vi "initialize Session Data.vi"(0 "Session in":refnum<class "SLSC Session.lvclass">, 11 "error in":errorcluster) -> (4 "Session out":refnum<class "SLSC Session.lvclass">, 15 "error out":errorcluster)   [LabVIEW 2015, in "SLSC Switch.lvlib" / "SLSC Session.lvclass"]
uses:
  SLSC Session.lvclass
  SLSC Session.lvclass/SLSC Session.ctl
  <vilib>/SLSC/Initialize Session without Resources.vi
  <userlib>/_Session Fwk/Session - Root.lvclass
  <vilib>/SLSC/SLSC.lvlib
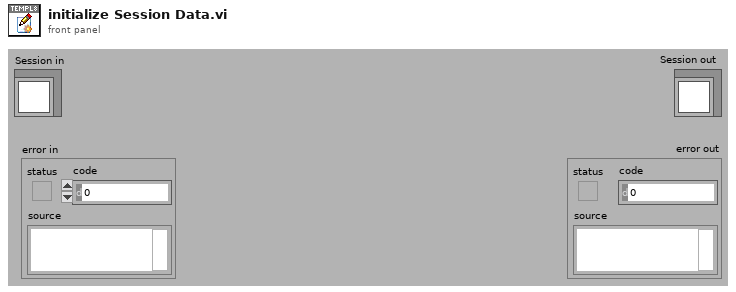
[diagram p1: front panel]
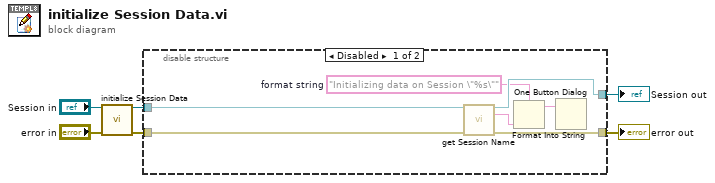
[diagram p0: block diagram]
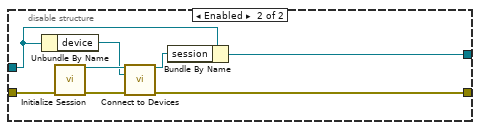
[diagram p2: hidden frame]
diagram:
  n1 = call-parent "initialize Session Data.vi"("OBJ - Session in"="Session in", "error in"="error in") -> ("OBJ - Session out"=w3:refnum<class "SLSC Session.lvclass">, "error out"=w1:errorcluster)  [unwired: 12 in]
  n2 = disable-structure shown="Disabled" {
    disable-tunnel: w3 -> [w13 w21]
    disable-tunnel: [w12 w20] -> w5
    disable-tunnel: w1 -> [w8 w15]
    disable-tunnel: [w7 w14] -> w6
    frame Disabled {
      w10 = "Initializing data on Session \"%s\""  # format string
      n3 = call <userlib>:"get Session Name.vi"("OBJ - Session in"=w13, "error in (no error)"=w8) -> ("OBJ - Session out"=w12:refnum<class "SLSC Session.lvclass">, "Session Name"=w11:string, "error out"=w7:errorcluster)  [unwired: 11 in]
      n4 = Format Into String(format string=w10, w11) -> (resulting string=w9:string)  [unwired: 2 in, 1 out]
      n5 = One Button Dialog(message=w9) -> ()  [unwired: 1 in, 1 out]
    }
    frame Enabled {
      n6 = Unbundle By Name(w21) -> ("device"=w17:refnum<k21>)
      n7 = call-poly <vilib>:"Initialize Session.vi"("error in (no error)"=w15) -> ("session out"=w19:refnum<k21>, "error out"=w18:errorcluster)  [unwired: 13 in]
      n8 = call <vilib>:"Connect to Devices.vi"("session in"=w19, "devices"=w17, "error in (no error)"=w18) -> ("session out"=w16:refnum<k21>, "error out"=w14:errorcluster)  [unwired: 11 in]
      n9 = Bundle By Name(cluster=w21, "session"=w16) -> (w20:refnum<class "SLSC Session.lvclass">)
    }
  }
  "error out" <- w6
  "Session out" <- w5
